vi "GUI - RPC File (V1.00).vi"(0 "Time Data IN":refnum<class "GSwFormDSP.lvclass">, 5 "error in (no error)":errorcluster, 7 "Application Name":string="GSwForm", 9 "State Queue":string[](array[string])=["SC: Initialize"], 11 "RPC File Path - READ":path, 13 "RPC File Path - WRITE":path) -> (14 "SubVI Time Data DUP":refnum<class "GSwFormDSP.lvclass">, 19 "error out":errorcluster)   [LabVIEW 2022 SP3, in "RPC.lvclass"]
uses:
  RPC.lvclass
  API/GSwFormDSP_class/GSwFormDSP.lvclass
  <vilib>/Utility/sysdir.llb/System Directory Type.ctl
  W:/projects/archives/23 Charette AI Group/SPWB/API/Generic Utilities_class/Generic Utilities.lvclass
  <vilib>/addons/_AddQ/G#Object/G#Object.lvclass
  API/Generic Utilities_class/Generic Utilities.lvclass
panel:
  in  "Task":enum32{"Monitor", "Settings"}(tab)
  out "Waveform Graph":waveform(dbl)[](graph)
  in  "READ - Select RPC File":bool
  in  "WRITE - Select RPC File":bool
  out "State History":string[](array[string])
  out "State Index":i32
  in  "Exit":bool
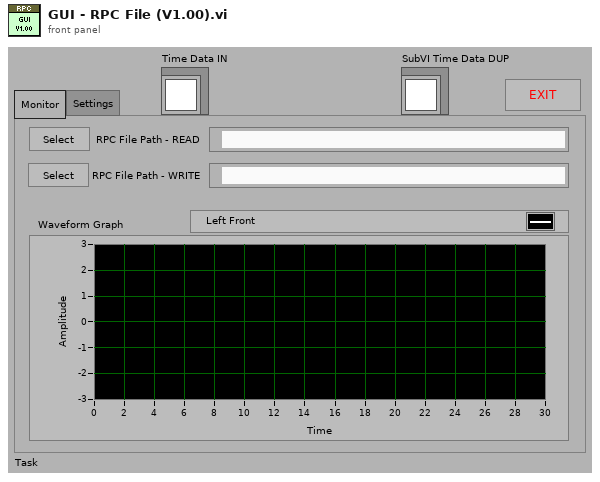
[diagram p1: front panel]
types:
  T1 = enum32{"Invalid", "Standard", "Closed", "Hidden", "Minimized", "Maximized"}
  T2 = typedef "System Directory Type.ctl" = i32
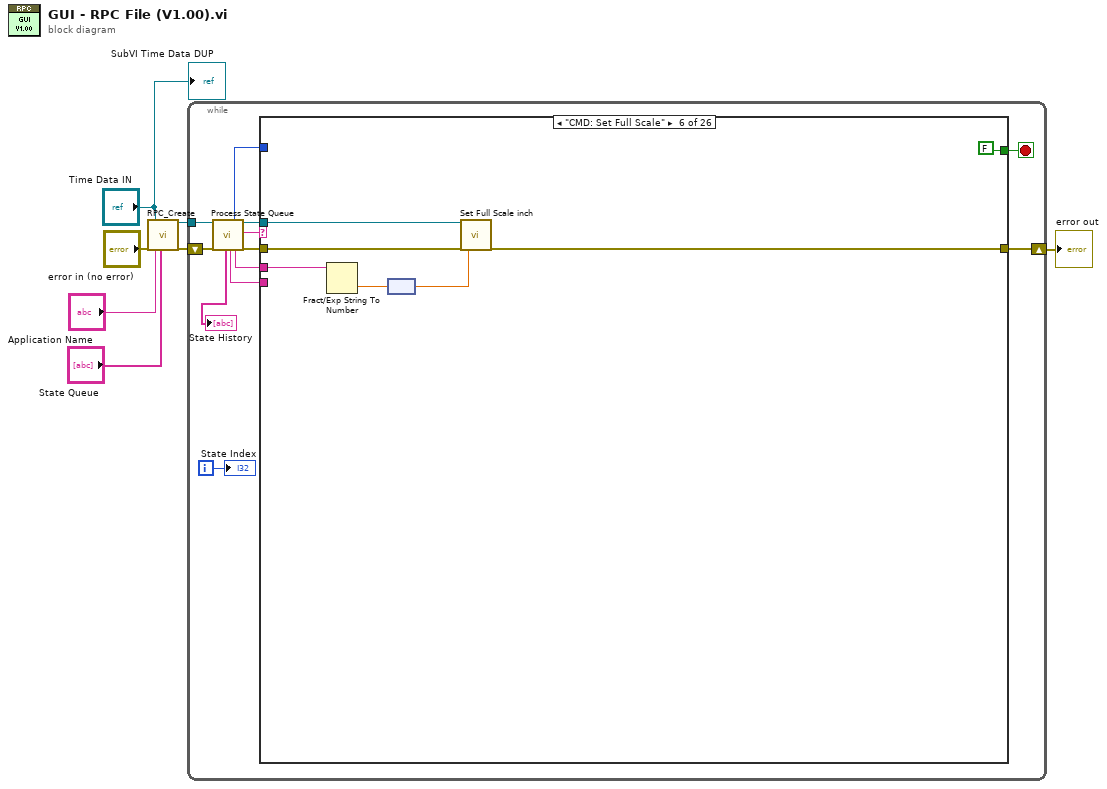
[diagram p0: block diagram]
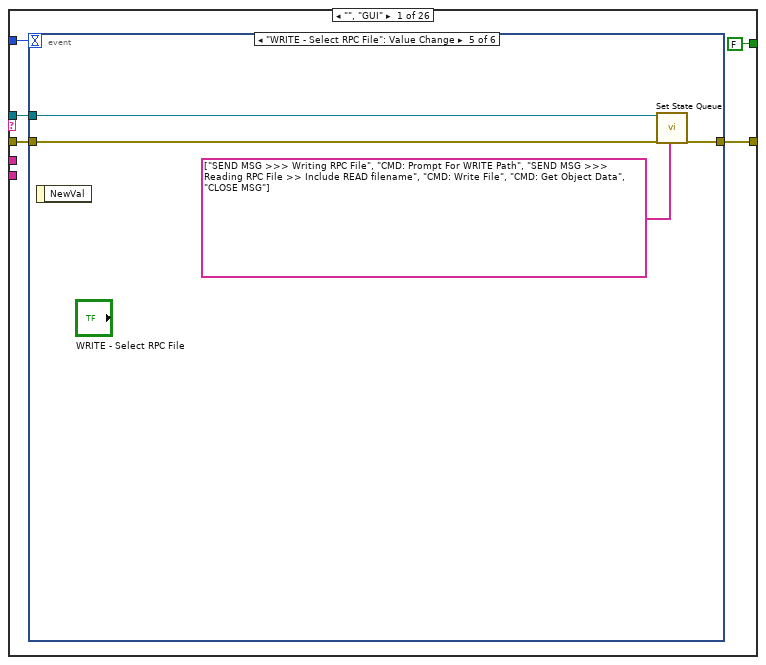
[diagram p2: hidden frame]
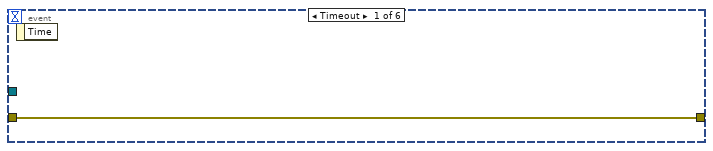
[diagram p3: hidden frame]
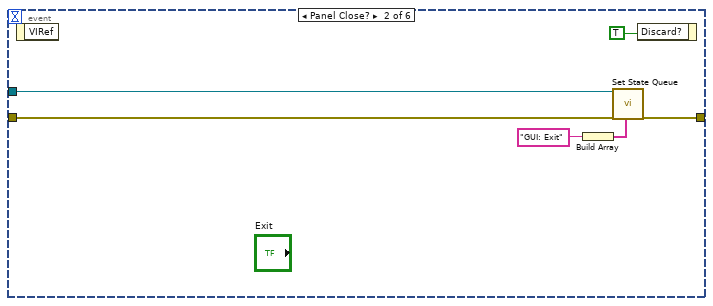
[diagram p4: hidden frame]
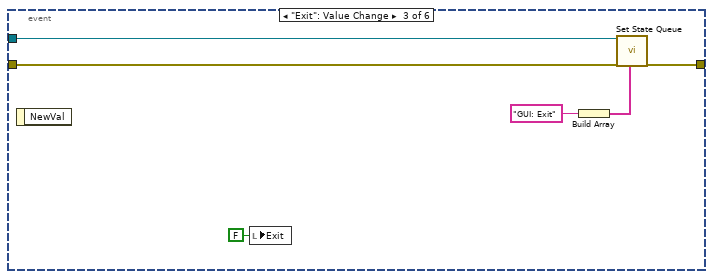
[diagram p5: hidden frame]
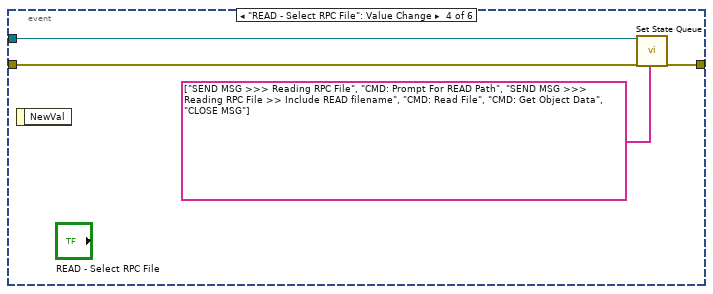
[diagram p6: hidden frame]
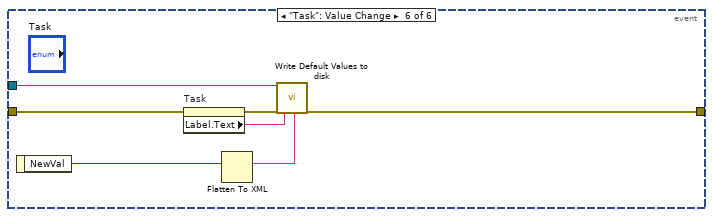
[diagram p7: hidden frame]
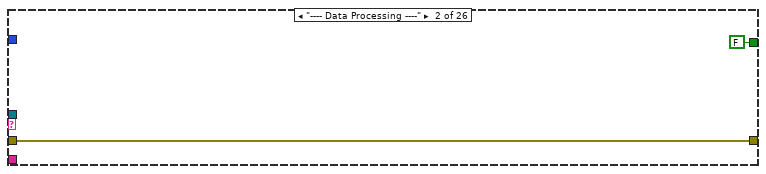
[diagram p8: hidden frame]
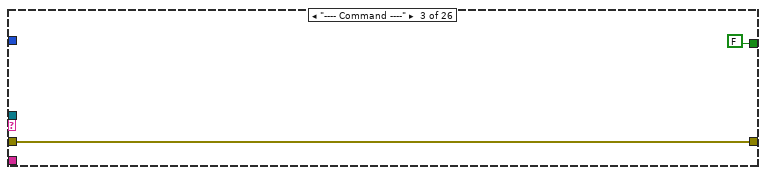
[diagram p9: hidden frame]
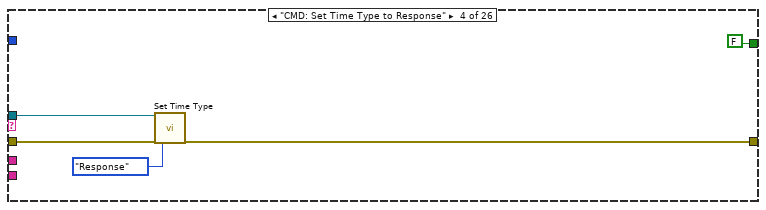
[diagram p10: hidden frame]
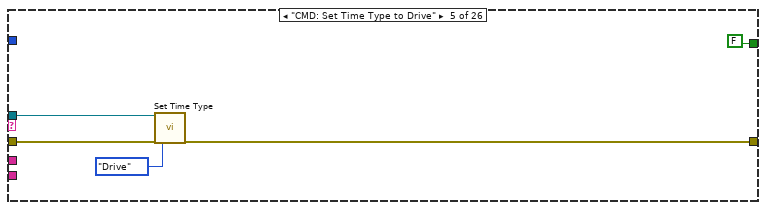
[diagram p11: hidden frame]
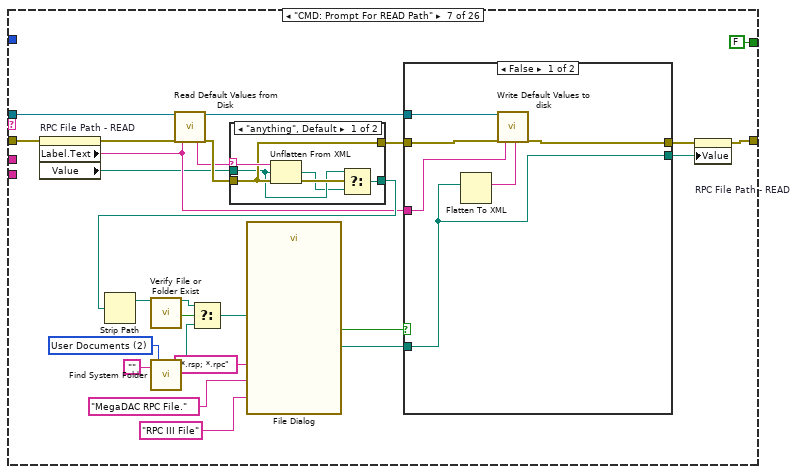
[diagram p12: hidden frame]
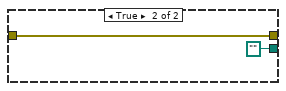
[diagram p13: hidden frame]
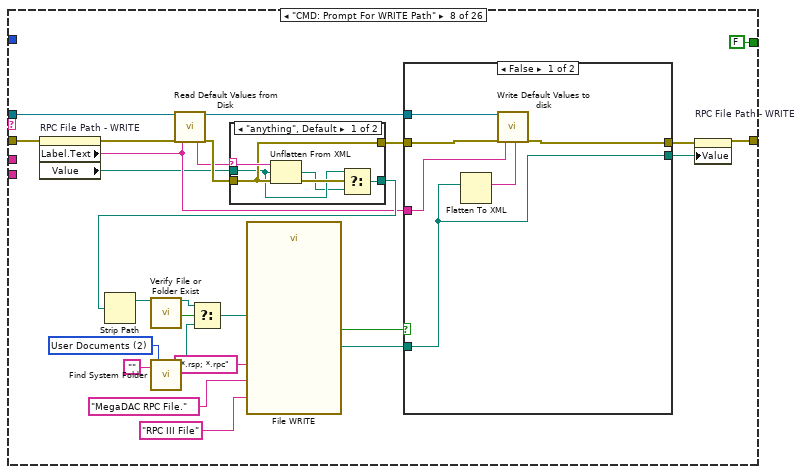
[diagram p15: hidden frame]
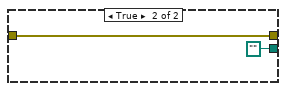
[diagram p16: hidden frame]
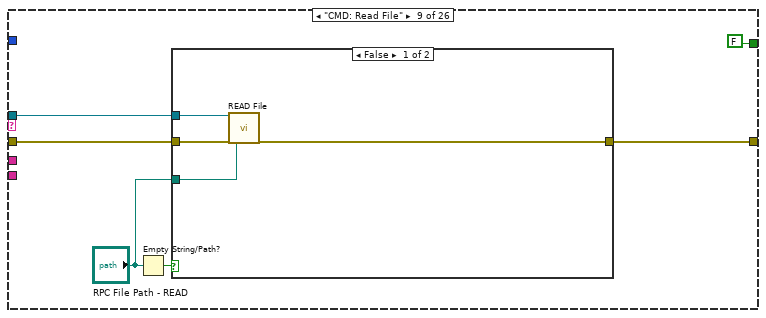
[diagram p18: hidden frame]
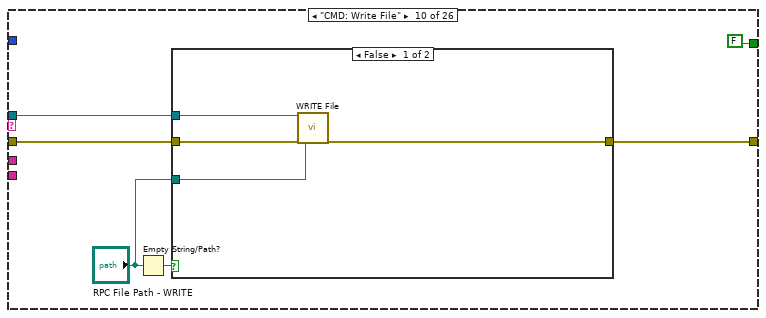
[diagram p20: hidden frame]
diagram:
  n1 = call "RPC_Create.vi"("error in (no error)"="error in (no error)", "Time Data IN"="Time Data IN", "Application Name"="Application Name", "State Queue"="State Queue") -> ("reference out"=w7:refnum<class "RPC.lvclass">, "error out"=w6:errorcluster)  [unwired: 14 in]
  n2 = while {
    shift-right: [w11] -> w2
    shift-left: w6 -> [w16]
    tunnel: w7 -> [w17]
    i -> [w18]
    stop <- w19 stop-if-true
    n3 = call "Process State Queue.vi"("reference in"=w17, "error in (no error)"=w16) -> ("State History"=→"State History":string[], "Additional Options"=w9:string, "Timeout"=w15:i32, "State Option"=w10:string, "reference out"=w14:refnum<class "RPC.lvclass">, "Current State"=w13:string, "error out"=w12:errorcluster)  [unwired: 10 in, 1 out]
    n4 = case shown="\"CMD: Set Full Scale\"" w13 {
      selector: w13 -> [_ _ _ _ _ _ _ _ _ _ _ _ _ _ _ _ _ _ _ _ _ _ w364 _ _ _]
      tunnel: w14 -> [w22 _ _ w60 w65 w72 w75 w117 w158 w169 w184 _ w192 _ w198 w228 _ w262 w281 w316 w346 _ _ _ _ w374]
      tunnel: [FALSE FALSE FALSE FALSE FALSE FALSE FALSE FALSE FALSE FALSE FALSE FALSE FALSE FALSE FALSE FALSE FALSE FALSE TRUE FALSE FALSE FALSE FALSE FALSE FALSE TRUE] -> w19
      tunnel: w15 -> [w23 _ _ _ _ _ _ _ _ _ _ _ _ _ _ _ _ _ _ _ _ _ _ _ _ _]
      tunnel: w10 -> [_ _ _ _ _ w69 _ _ _ _ _ _ _ _ w199 w225 _ _ _ w325 _ _ _ _ _ _]
      tunnel: w12 -> [w21 w53 w55 w59 w64 w71 w82 w124 w161 w172 w185 w187 w191 w194 w196 w227 w248 w259 w278 w315 w347 w360 w362 w367 w370 w373]
      tunnel: [w20 w53 w55 w58 w63 w70 w77 w119 w160 w171 w181 w187 w190 w194 w197 w226 w248 w250 w277 w313 w343 w360 w362 errorcluster {"status"=FALSE, "code"=0, "source"=""} ("error out") w370 w372] -> w11
      tunnel: w9 -> [_ _ _ _ _ _ _ _ _ _ _ _ _ _ _ _ _ _ _ w311 _ _ _ _ _ _]
      frame "", "GUI" {
        n5 = event shown="[4] \"WRITE - Select RPC File\": Value Change" {
          selector: _ -> [_ _ _ _ _ _]
          dyn-events: _ -> [_ _ _ _ _ _]
          timeout: w23 -> [_ _ _ _ _ _]
          tunnel: w22 -> [_ w29 w35 w40 w44 w51]
          tunnel: w21 -> [w25 w28 w33 w39 w43 w48]
          tunnel: [w25 w27 w34 w41 w45 w46] -> w20
          event Timeout {
            n6 = event-data() -> ()  [unwired: 1 in, 1 out]
          }
          event Panel Close? {
            n7 = event-data() -> ()  [unwired: 1 in, 1 out]
            n8 = Build Array("GUI: Exit") -> (w26:string[])
            n9 = call "Set State Queue.vi"("reference in"=w29, "error in (no error)"=w28, "State Queue"=w26) -> ("error out"=w27:errorcluster)  [unwired: 15 in, 1 out]
            n10 = event-data("Discard?"=TRUE) -> ()  [unwired: 1 in, 1 out]
          }
          event "Exit": Value Change {
            n11 = event-data() -> ()  [unwired: 1 in, 1 out]
            n12 = local write "Exit"(FALSE ("Exit")) -> ()
            n13 = Build Array("GUI: Exit") -> (w32:string[])
            n14 = call "Set State Queue.vi"("reference in"=w35, "error in (no error)"=w33, "State Queue"=w32) -> ("error out"=w34:errorcluster)  [unwired: 15 in, 1 out]
          }
          event "READ - Select RPC File": Value Change {
            n15 = event-data() -> ()  [unwired: 1 in, 1 out]
            n16 = call "Set State Queue.vi"("reference in"=w40, "error in (no error)"=w39, "State Queue"=string[] ["SEND MSG >>> Reading RPC File", "CMD: Prompt For READ Path", "SEND MSG >>> Reading RPC File >> Include READ filename", "CMD: Read File", "CMD: Get Object Data", "CLOSE MSG"]) -> ("error out"=w41:errorcluster)  [unwired: 15 in, 1 out]
          }
          event "WRITE - Select RPC File": Value Change {
            n17 = event-data() -> ()  [unwired: 1 in, 1 out]
            n18 = call "Set State Queue.vi"("reference in"=w44, "error in (no error)"=w43, "State Queue"=string[] ["SEND MSG >>> Writing RPC File", "CMD: Prompt For WRITE Path", "SEND MSG >>> Reading RPC File >> Include READ filename", "CMD: Write File", "CMD: Get Object Data", "CLOSE MSG"]) -> ("error out"=w45:errorcluster)  [unwired: 15 in, 1 out]
          }
          event "Task": Value Change {
            n19 = event-data() -> ("NewVal"=w52:enum32{"Monitor", "Settings"})  [unwired: 1 in]
            n20 = property on="Task" class="TabCtl (strict)"(error in=w48) -> (error out=w47:errorcluster, "Label.Text"=w50:string)  [unwired: 1 in, 1 out]
            n21 = Flatten To XML(6:w52) -> (2:w49:string)
            n22 = call-dynamic "Write Default Values to disk.vi"("reference in"=w51, "error in (no error)"=w47, "Control Label"=w50, "Value (XML String)"=w49) -> ("error out"=w46:errorcluster)  [unwired: 14 in, 1 out]
          }
        }
      }
      frame "---- Data Processing ----" {
      }
      frame "---- Command ----" {
      }
      frame "CMD: Set Time Type to Response" {
        n23 = call "Set Time Type.vi"("reference in"=w60, "error in (no error)"=w59, "Time Type"=enum16{"Response", "Drive"}."Response") -> ("error out"=w58:errorcluster)  [unwired: 15 in, 1 out]
      }
      frame "CMD: Set Time Type to Drive" {
        n24 = call "Set Time Type.vi"("reference in"=w65, "error in (no error)"=w64, "Time Type"=enum16{"Response", "Drive"}."Drive") -> ("error out"=w63:errorcluster)  [unwired: 15 in, 1 out]
      }
      frame "CMD: Set Full Scale" {
        n25 = Fract/Exp String To Number(string=w69) -> (number=w68:dbl)  [unwired: 3 in, 1 out]
        n26 = node(w68) -> (w67:dbl[unit])
        n27 = call "Set Full Scale inch.vi"("reference in"=w72, "error in (no error)"=w71, "Full Scale"=w67) -> ("error out"=w70:errorcluster)  [unwired: 15 in, 1 out]
      }
      frame "CMD: Prompt For READ Path" {
        w89 = T2 2 items=["User Home"=0, "User Desktop"=1, "User Documents"=2, "User Application Data"=3, "User Preferences"=4, "User Temporary"=5, "Public Documents"=6, "Public Application Data"=7, "Public Preferences"=8, "Public Cache"=13, "System Core Libraries"=9, "System Installed Libraries"=10, "Application Files"=11, "Boot Volume Root"=12] ("system directory type")
        n28 = property on="RPC File Path - READ" class="Path"(error in=w82) -> (error out=w81:errorcluster, "Label.Text"=w80:string, "Value"=w79:path)  [unwired: 1 in, 1 out]
        n29 = call "Find System Folder.vi"("Application Name"="", "system directory type"=w89) -> ("System Folder"=w90:path)  [unwired: 16 in, 1 out]
        n30 = call-dynamic "Read Default Values from Disk.vi"("reference in"=w75, "error in (no error)"=w81, "Control Label"=w80) -> ("Value (XML String)"=w74:string, "reference out"=w97:refnum<class "RPC.lvclass">, "error out"=w83:errorcluster)  [unwired: 14 in]
        n31 = case shown="\"anything\", Default" w74 {
          selector: w74 -> [w113 _]
          tunnel: [w108 w115] -> w84
          tunnel: w79 -> [w110 w115]
          tunnel: w83 -> [w111 w114]
          tunnel: [w111 w114] -> w96
          frame "anything", Default {
            n32 = Unflatten From XML(xml string=w113, type=w110, error in (no error)=w111) -> (value=w109:path, error out=w112:errorcluster)
            n33 = Select(t=w110, s=w112, f=w109) -> (s? t:f=w108:path)
          }
          frame "" {
            # "Either the file was not found or there was some error"
          }
        }
        n34 = Strip Path(path=w84) -> (stripped path=w85:path)  [unwired: 1 out]
        n35 = call "Verify File or Folder Exist.vi"("path"=w85) -> ("dup path"=w87:path, "file or folder exists?"=w86:bool)  [unwired: 16 in, 1 out]
        n36 = Select(t=w87, s=w86, f=w90) -> (s? t:f=w88:path)
        n37 = call "File Dialog"("start path"=w88, "button label"="RPC III File", "pattern (all files)"="*.rsp; *.rpc", "pattern label"="MegaDAC RPC File.") -> ("selected path"=w98:path, "cancelled"=w95:bool)  [unwired: 8 in, 2 out]
        n38 = case shown="False" w95 {
          tunnel: [w101 w107] -> w78
          tunnel: w96 -> [w102 w107]
          tunnel: [w100 path ""] -> w76
          tunnel: w97 -> [w104 _]
          tunnel: w80 -> [w103 _]
          tunnel: w98 -> [w100 _]
          frame False {
            n39 = Flatten To XML(6:w100) -> (2:w105:string)
            n40 = call-dynamic "Write Default Values to disk.vi"("reference in"=w104, "error in (no error)"=w102, "Control Label"=w103, "Value (XML String)"=w105) -> ("error out"=w101:errorcluster)  [unwired: 14 in, 1 out]
          }
          frame True {
          }
        }
        n41 = property on="RPC File Path - READ" class="Path"(error in=w78, "Value"=w76) -> (error out=w77:errorcluster)  [unwired: 1 in, 1 out]
      }
      frame "CMD: Prompt For WRITE Path" {
        w131 = T2 2 items=["User Home"=0, "User Desktop"=1, "User Documents"=2, "User Application Data"=3, "User Preferences"=4, "User Temporary"=5, "Public Documents"=6, "Public Application Data"=7, "Public Preferences"=8, "Public Cache"=13, "System Core Libraries"=9, "System Installed Libraries"=10, "Application Files"=11, "Boot Volume Root"=12] ("system directory type")
        n42 = property on="RPC File Path - WRITE" class="Path"(error in=w124) -> (error out=w123:errorcluster, "Label.Text"=w122:string, "Value"=w121:path)  [unwired: 1 in, 1 out]
        n43 = call "Find System Folder.vi"("Application Name"="", "system directory type"=w131) -> ("System Folder"=w132:path)  [unwired: 16 in, 1 out]
        n44 = call-dynamic "Read Default Values from Disk.vi"("reference in"=w117, "error in (no error)"=w123, "Control Label"=w122) -> ("Value (XML String)"=w116:string, "reference out"=w139:refnum<class "RPC.lvclass">, "error out"=w125:errorcluster)  [unwired: 14 in]
        n45 = case shown="\"anything\", Default" w116 {
          selector: w116 -> [w155 _]
          tunnel: [w150 w157] -> w126
          tunnel: w121 -> [w152 w157]
          tunnel: w125 -> [w153 w156]
          tunnel: [w153 w156] -> w138
          frame "anything", Default {
            n46 = Unflatten From XML(xml string=w155, type=w152, error in (no error)=w153) -> (value=w151:path, error out=w154:errorcluster)
            n47 = Select(t=w152, s=w154, f=w151) -> (s? t:f=w150:path)
          }
          frame "" {
            # "Either the file was not found or there was some error"
          }
        }
        n48 = Strip Path(path=w126) -> (stripped path=w127:path)  [unwired: 1 out]
        n49 = call "Verify File or Folder Exist.vi"("path"=w127) -> ("dup path"=w129:path, "file or folder exists?"=w128:bool)  [unwired: 16 in, 1 out]
        n50 = Select(t=w129, s=w128, f=w132) -> (s? t:f=w130:path)
        n51 = call "File WRITE"("start path"=w130, "button label"="RPC III File", "pattern (all files)"="*.rsp; *.rpc", "pattern label"="MegaDAC RPC File.") -> ("selected path"=w140:path, "cancelled"=w137:bool)  [unwired: 8 in, 2 out]
        n52 = case shown="False" w137 {
          tunnel: [w143 w149] -> w120
          tunnel: w138 -> [w144 w149]
          tunnel: [w142 path ""] -> w118
          tunnel: w139 -> [w146 _]
          tunnel: w122 -> [w145 _]
          tunnel: w140 -> [w142 _]
          frame False {
            n53 = Flatten To XML(6:w142) -> (2:w147:string)
            n54 = call-dynamic "Write Default Values to disk.vi"("reference in"=w146, "error in (no error)"=w144, "Control Label"=w145, "Value (XML String)"=w147) -> ("error out"=w143:errorcluster)  [unwired: 14 in, 1 out]
          }
          frame True {
          }
        }
        n55 = property on="RPC File Path - WRITE" class="Path"(error in=w120, "Value"=w118) -> (error out=w119:errorcluster)  [unwired: 1 in, 1 out]
      }
      frame "CMD: Read File" {
        n56 = Empty String/Path?(string/path="RPC File Path - READ") -> (empty?=w162:bool)
        n57 = case shown="False" w162 {
          tunnel: w161 -> [w165 w168]
          tunnel: [w166 w168] -> w160
          tunnel: "RPC File Path - READ" -> [w167 _]
          tunnel: w158 -> [w164 _]
          frame False {
            n58 = call "READ File.vi"("reference in"=w164, "error in (no error)"=w165, "MegaDAC RPC File (*.rsp)"=w167) -> ("error out"=w166:errorcluster)  [unwired: 15 in, 1 out]
          }
          frame True {
          }
        }
      }
      frame "CMD: Write File" {
        n59 = Empty String/Path?(string/path="RPC File Path - WRITE") -> (empty?=w173:bool)
        n60 = case shown="False" w173 {
          tunnel: w172 -> [w178 w179]
          tunnel: [w176 w179] -> w171
          tunnel: "RPC File Path - WRITE" -> [w175 _]
          tunnel: w169 -> [w177 _]
          frame False {
            n61 = call "WRITE File.vi"("reference in"=w177, "error in (no error)"=w178, "MegaDAC RPC File (*.rsp)"=w175) -> ("error out"=w176:errorcluster)  [unwired: 15 in, 1 out]
          }
          frame True {
          }
        }
      }
      frame "CMD: Get Object Data" {
        n62 = call "Get Obj Data.vi"("reference in"=w184, "error in (no error)"=w185) -> ("Time Data"=w183:refnum<class "GSwFormDSP.lvclass">, "error out"=w182:errorcluster)  [unwired: 15 in, 1 out]
        n63 = call-dynamic "Get - wForms.vi"("reference in"=w183, "error in (no error)"=w182) -> ("wForms"=→"Waveform Graph":waveform(dbl)[], "error out"=w181:errorcluster)  [unwired: 14 in, 2 out]
      }
      frame "---- Scripts ----" {
      }
      frame "SC: Initialize" {
        n64 = call "Set State Queue.vi"("reference in"=w192, "error in (no error)"=w191, "State Queue"=string[] ["GUI: Initialize Ref", "CTRL >>> Task Tab", "FP >>> Open"] ("State Queue OUT")) -> ("error out"=w190:errorcluster)  [unwired: 15 in, 1 out]
      }
      frame "---- Front Panel Mgmt ----" {
      }
      frame "CTRL" {
        n65 = case shown="\"Task Tab\"" w199 {
          selector: w199 -> [w204 _]
          tunnel: [w202 w208] -> _
          tunnel: w198 -> [w202 w213]
          tunnel: [w201 w207] -> w197
          tunnel: w196 -> [w201 w211]
          frame "unknown", Default {
            n66 = Concatenate Strings("The following control name is unrecognized:\n", w204) -> (w203:string)
            n67 = One Button Dialog(message=w203) -> ()  [unwired: 1 in, 1 out]
          }
          frame "Task Tab" {
            n68 = property on="Task" class="TabCtl (strict)"(error in=w211) -> (error out=w212:errorcluster, "Label.Text"=w210:string, "Value"=w215:enum32{"Monitor", "Settings"})  [unwired: 1 in, 1 out]
            n69 = call-dynamic "Read Default Values from Disk.vi"("reference in"=w213, "error in (no error)"=w212, "Control Label"=w210) -> ("Value (XML String)"=w206:string, "reference out"=w208:refnum<class "RPC.lvclass">, "error out"=w209:errorcluster)  [unwired: 14 in]
            n70 = case shown="\"\"" w206 {
              selector: w206 -> [w222 _]
              tunnel: [w217 w224] -> w216
              tunnel: w215 -> [w219 w224]
              tunnel: w209 -> [w220 w223]
              tunnel: [w220 w223] -> w214
              frame "anything", Default {
                n71 = Unflatten From XML(xml string=w222, type=w219, error in (no error)=w220) -> (value=w218:enum32{"Monitor", "Settings"}, error out=w221:errorcluster)
                n72 = Select(t=w219, s=w221, f=w218) -> (s? t:f=w217:enum32{"Monitor", "Settings"})
              }
              frame "" {
                # "Either the file was not found or there was some error"
              }
            }
            n73 = property on="Task" class="TabCtl (strict)"(error in=w214, "Value"=w216) -> (error out=w207:errorcluster)  [unwired: 1 in, 1 out]
          }
        }
      }
      frame "FP" {
        n74 = case shown="\"Open\"" w225 {
          selector: w225 -> [w230 _]
          tunnel: w228 -> [_ w238]
          tunnel: w227 -> [w231 w237]
          tunnel: [w231 w234] -> w226
          frame "unknown", Default {
            n75 = Concatenate Strings("The following FP Command name is unrecognized:\n", w230) -> (w232:string)
            n76 = One Button Dialog(message=w232) -> ()  [unwired: 1 in, 1 out]
          }
          frame "Open" {
            n77 = call-dynamic "Get VI Ref.vi"("reference in"=w238, "error in (no error)"=w237) -> ("GUI VI Ref"=w235:refnum<vi>, "error out"=w236:errorcluster)  [unwired: 14 in, 2 out]
            n78 = property class="VI"(reference=w235, error in=w236) -> (reference out=w240:refnum<vi>, error out=w241:errorcluster, "Front Panel.Open"=w239:bool)
            n79 = case shown="False" w239 {
              tunnel: [w244 w247] -> w234
              tunnel: w241 -> [w243 w247]
              tunnel: w240 -> [w242 _]
              frame False {
                n80 = invoke class="VI" method="FP.Open"(reference=w242, error in=w243, "Activate"=TRUE, "State"=T1."Standard") -> (error out=w244:errorcluster)  [unwired: 1 in, 4 out]
              }
              frame True {
              }
            }
          }
        }
      }
      frame "---- GUI Functions ----" {
      }
      frame "GUI: Initialize Ref" {
        n81 = control-ref of="GUI Reference"() -> (w258:refnum<vi>)
        n82 = call "Set VI Ref.vi"("reference in"=w262, "error in (no error)"=w259, "GUI VI Ref"=w258) -> ("reference out"=w261:refnum<class "RPC.lvclass">, "error out"=w257:errorcluster)  [unwired: 15 in]
        n83 = call "Set Close Panel (Yes or No).vi"("reference in"=w261, "error in (no error)"=w257) -> ("reference out"=w260:refnum<class "RPC.lvclass">, "error out"=w256:errorcluster)  [unwired: 16 in]
        n84 = call "Set Message Window Ref.vi"("reference in"=w260, "error in (no error)"=w256) -> ("reference out"=w254:refnum<class "RPC.lvclass">, "error out"=w255:errorcluster)  [unwired: 16 in]
        n85 = call "Get - Time Data OBJ State.vi"("reference in"=w254, "error in (no error)"=w255) -> ("New Time Data Obj?"=w253:bool, "reference out"=w252:refnum<class "RPC.lvclass">, "error out"=w251:errorcluster)  [unwired: 15 in]
        n86 = case shown="True" w253 {
          tunnel: w252 -> [_ w270]
          tunnel: w251 -> [w264 w269]
          tunnel: [w264 w265] -> w250
          frame False {
          }
          frame True {
            n87 = call "Get Obj Data.vi"("reference in"=w270, "error in (no error)"=w269) -> ("Time Data"=w267:refnum<class "GSwFormDSP.lvclass">, "error out"=w266:errorcluster)  [unwired: 15 in, 1 out]
            n88 = call "Set - wForms.vi"("reference in"=w267, "error in (no error)"=w266, "Init wForms"=TRUE) -> ("error out"=w265:errorcluster)  [unwired: 15 in, 1 out]
          }
        }
      }
      frame "GUI: Exit" {
        n89 = call-dynamic "Get Message Window Ref.vi"("reference in"=w281, "error in (no error)"=w278) -> ("reference out"=w280:refnum<class "RPC.lvclass">, "Msg Win Ref"=w276:refnum<vi>, "error out"=w279:errorcluster)  [unwired: 15 in]
        n90 = call-dynamic "Get VI Ref.vi"("reference in"=w280, "error in (no error)"=w279) -> ("reference out"=w285:refnum<class "RPC.lvclass">, "GUI VI Ref"=w283:refnum<vi>, "error out"=w284:errorcluster)  [unwired: 14 in, 1 out]
        n91 = call-dynamic "Get Close Panel (Yes or No).vi"("reference in"=w285, "error in (no error)"=w284) -> ("Close Panel?"=w286:bool, "reference out"=w275:refnum<class "RPC.lvclass">, "error out"=w273:errorcluster)  [unwired: 15 in]
        n92 = call "Get - Time Data OBJ State.vi"("reference in"=w275, "error in (no error)"=w273) -> ("New Time Data Obj?"=w271:bool, "reference out"=w274:refnum<class "RPC.lvclass">, "error out"=w272:errorcluster)  [unwired: 15 in]
        n93 = call-dynamic "Destroy.vi"("reference in"=w274, "error in (no error)"=w272) -> ("error out"=w290:errorcluster)  [unwired: 16 in, 1 out]
        n94 = case shown="True" w271 {
          tunnel: w290 -> [w292 w294]
          tunnel: [w292 w293] -> w282
          frame False {
          }
          frame True {
            n95 = call <vilib>:"GarbageCollector.vi"("error in (no error)"=w294) -> ("error out"=w293:errorcluster)  [unwired: 16 in, 2 out]
          }
        }
        n96 = Close Reference(reference=w276, error in (no error)=w282) -> (error out=w289:errorcluster)
        n97 = case shown="True" w286 {
          tunnel: w289 -> [w296 w300]
          tunnel: [w296 w299] -> w287
          tunnel: [w295 w298] -> w288
          tunnel: w283 -> [w295 w297]
          frame False {
          }
          frame True {
            n98 = property class="VI"(reference=w297, error in=w300) -> (reference out=w302:refnum<vi>, error out=w301:errorcluster, "Front Panel.Open"=w303:bool)
            n99 = case shown="True" w303 {
              tunnel: [w305 w309] -> w299
              tunnel: w301 -> [w305 w308]
              tunnel: w302 -> [w304 w307]
              tunnel: [w304 w306] -> w298
              frame False {
              }
              frame True {
                n100 = invoke class="VI" method="FP.Close"(reference=w307, error in=w308) -> (reference out=w306:refnum<vi>, error out=w309:errorcluster)  [unwired: 1 in, 1 out]
              }
            }
          }
        }
        n101 = Close Reference(reference=w288, error in (no error)=w287) -> (error out=w277:errorcluster)
      }
      frame "SEND MSG" {
        n102 = call-dynamic "Get Message Window Ref.vi"("reference in"=w316, "error in (no error)"=w315) -> ("Msg Win Ref"=w312:refnum<vi>, "error out"=w314:errorcluster)  [unwired: 15 in, 1 out]
        n103 = case shown="\"Include READ filename\"" w311 {
          tunnel: ["" w328] -> w310
          frame "None", Default {
          }
          frame "Include READ filename" {
            n104 = local read "RPC File Path - READ"() -> (w331:path)
            n105 = Path To String(path=w331) -> (string=w330:string)
            n106 = Concatenate Strings("\r", w330) -> (w328:string)
          }
        }
        n107 = property class="VI"(reference=w312, error in=w314) -> (reference out=w318:refnum<vi>, error out=w317:errorcluster, "Front Panel.Open"=w319:bool)
        n108 = case shown="False" w319 {
          tunnel: [w338 w342] -> w321
          tunnel: w317 -> [w333 w342]
          tunnel: w318 -> [w335 w341]
          tunnel: [w337 w341] -> w320
          frame False {
            w336 = FALSE ("Wait Until Done")
            n109 = invoke class="VI" method="Run VI"(reference=w335, error in=w333, "Wait until done"=w336, "Auto Dispose Ref"=w336) -> (reference out=w334:refnum<vi>, error out=w332:errorcluster)  [unwired: 1 in, 3 out]
            n110 = invoke class="VI" method="FP.Open"(reference=w334, error in=w332, "Activate"=TRUE, "State"=T1."Standard") -> (reference out=w337:refnum<vi>, error out=w338:errorcluster)  [unwired: 1 in, 3 out]
          }
          frame True {
          }
        }
        n111 = Concatenate Strings("\r\n", w325, w310) -> (w324:string)
        n112 = invoke class="VI" method="Ctrl Val.Set"(reference=w320, error in=w321, "Control Name"="Message", "Value"=w324) -> (error out=w313:errorcluster)  [unwired: 1 in, 4 out]
      }
      frame "CLOSE MSG" {
        n113 = call-dynamic "Get Message Window Ref.vi"("reference in"=w346, "error in (no error)"=w347) -> ("Msg Win Ref"=w344:refnum<vi>, "error out"=w345:errorcluster)  [unwired: 15 in, 1 out]
        n114 = property class="VI"(reference=w344, error in=w345) -> (reference out=w351:refnum<vi>, error out=w352:errorcluster, "Front Panel.Open"=w350:bool)
        n115 = case shown="True" w350 {
          tunnel: [w355 w359] -> w349
          tunnel: w352 -> [w355 w358]
          tunnel: w351 -> [w354 w357]
          tunnel: [w354 w356] -> w348
          frame False {
          }
          frame True {
            n116 = invoke class="VI" method="FP.Close"(reference=w357, error in=w358) -> (reference out=w356:refnum<vi>, error out=w359:errorcluster)  [unwired: 1 in, 1 out]
          }
        }
        n117 = invoke class="VI" method="Abort VI"(reference=w348, error in=w349) -> (error out=w343:errorcluster)  [unwired: 1 in, 2 out]
      }
      frame "---- Miscelleneous ----" {
      }
      frame "unknown", Default {
        n118 = Concatenate Strings("The following state is unrecognized?\n", w364) -> (w363:string)
        n119 = One Button Dialog(message=w363) -> ()  [unwired: 1 in, 1 out]
      }
      frame "Error" {
        n120 = call <vilib>:"General Error Handler.vi"("error in (no error)"=w367) -> ()  [unwired: 10 in, 5 out]
      }
      frame "Next" {
        # "This is an empty case used so the queue does NOT stop if there is an empty string between two valid states!"
      }
      frame "Quit" {
        # "This is the case used to simply exit when this GUI is used as a SubVI!"
        n121 = call-dynamic "Destroy.vi"("reference in"=w374, "error in (no error)"=w373) -> ("error out"=w372:errorcluster)  [unwired: 16 in, 1 out]
      }
    }
    "State Index" <- w18
  }
  "error out" <- w2
  "SubVI Time Data DUP" <- "Time Data IN"
